vi "Test_IMU_DMP.vi"() -> ()   [LabVIEW 2014]
uses:
  <userlib>/UCSD Robotics Lab/Robotics-Cape/LV/libroboticscape.lvlib
panel:
  out "State":T1(ring)
  out "Timing Block":T2 {"Actual Hz" format="%#_3g"; "Dt" format="%#_4g"; "Average Hz" format="%#_4g"}
  out "Quarternion":T3
  in  "Quarternion On/Off":bool
  in  "Input Prior to Start":T4={"orientation"=112, "IMU_sample_rate "=100, "dmp_interrupt_priority"=98, "Enable Magnetometer"=FALSE} {"dmp_interrupt_priority" min=1 max=99 step=1; "IMU_sample_rate" min=4 max=200; "orientation" items=["ORIENTATION_Z_UP"=136, "ORIENTATION_Z_DOWN"=396, "ORIENTATION_X_UP"=14, "ORIENTATION_X_DOWN"=266, "ORIENTATION_Y_UP"=112, "ORIENTATION_Y_DOWN"=336, "ORIENTATION_X_FORWARD"=133, "ORIENTATION_X_BACK"=161]}
  out "Gryo":T5
  out "Accel":T6
  out "Tait Bryan":T7
  in  "Gyro On/Off":bool
  in  "Accel On/Off":bool
  in  "TaitBryan On/Off":bool
  in  "Compass On/Off":bool
  out "Compass":T8
  in  "stop":bool
  # "Always stop the VI using the rectangular STOP button below, never with the round stopsign (Abort)"
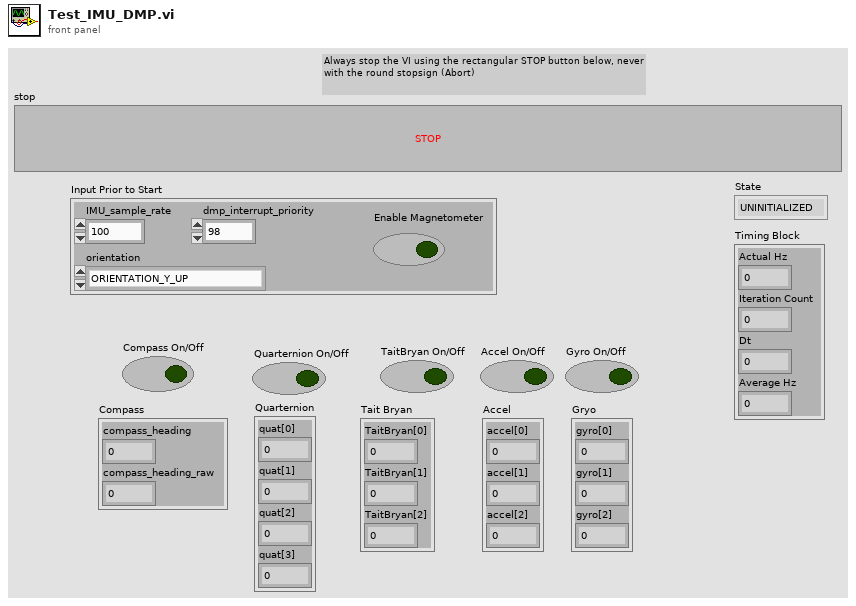
[diagram p1: front panel]
types:
  T1 = enum16{"UNINITIALIZED", "RUNNING", "PAUSED", "EXITING"}
  T2 = cluster{"Actual Hz":dbl, "Iteration Count":dbl, "Dt":dbl, "Average Hz":dbl}
  T3 = cluster{"quat[0]":sgl, "quat[1]":sgl, "quat[2]":sgl, "quat[3]":sgl}
  T4 = cluster{"orientation":u32, "IMU_sample_rate ":i32, "dmp_interrupt_priority":i32, "Enable Magnetometer":bool}
  T5 = cluster{"gyro[0]":sgl, "gyro[1]":sgl, "gyro[2]":sgl}
  T6 = cluster{"accel[0]":sgl, "accel[1]":sgl, "accel[2]":sgl}
  T7 = cluster{"TaitBryan[0]":dbl, "TaitBryan[1]":dbl, "TaitBryan[2]":dbl}
  T8 = cluster{"compass_heading":sgl, "compass_heading_raw":sgl}
  T9 = cluster{"accel[0]":sgl, "accel[1]":sgl, "accel[2]":sgl, "gyro[0]":sgl, "gyro[1]":sgl, "gyro[2]":sgl, "mag[0]":sgl, "mag[1]":sgl, "mag[2]":sgl, "temp":sgl, "raw_gyro[0]":i16, "raw_gyro[1]":i16, "raw_gyro[2]":i16, "raw_accel[0]":i16, "raw_accel[1]":i16, "raw_accel[2]":i16, "accel_to_ms2":sgl, "gyro_to_degs":sgl, "dmp_quat[0]":sgl, "dmp_quat[1]":sgl, "dmp_quat[2]":sgl, "dmp_quat[3]":sgl, "dmp_TaitBryan[0]":sgl, "dmp_TaitBryan[1]":sgl, "dmp_TaitBryan[2]":sgl, "fused_quat[0]":sgl, "fused_quat[1]":sgl, "fused_quat[2]":sgl, "fused_quat[3]":sgl, "fused_TaitBryan[0]":sgl, "fused_TaitBryan[1]":sgl, "fused_TaitBryan[2]":sgl, "compass_heading":sgl, "compass_heading_raw":sgl}
  T10 = enum16{"UNINITIALIZED", "RUNING", "PAUSED", "EXITING"}
  T11 = cluster{"fused_quat[0]":sgl, "fused_quat[1]":sgl, "fused_quat[2]":sgl, "fused_quat[3]":sgl}
  T12 = cluster{"fused_TaitBryan[0]":sgl, "fused_TaitBryan[1]":sgl, "fused_TaitBryan[2]":sgl}
  T13 = cluster{"fused_TaitBryan[0]":dbl, "fused_TaitBryan[1]":dbl, "fused_TaitBryan[2]":dbl}
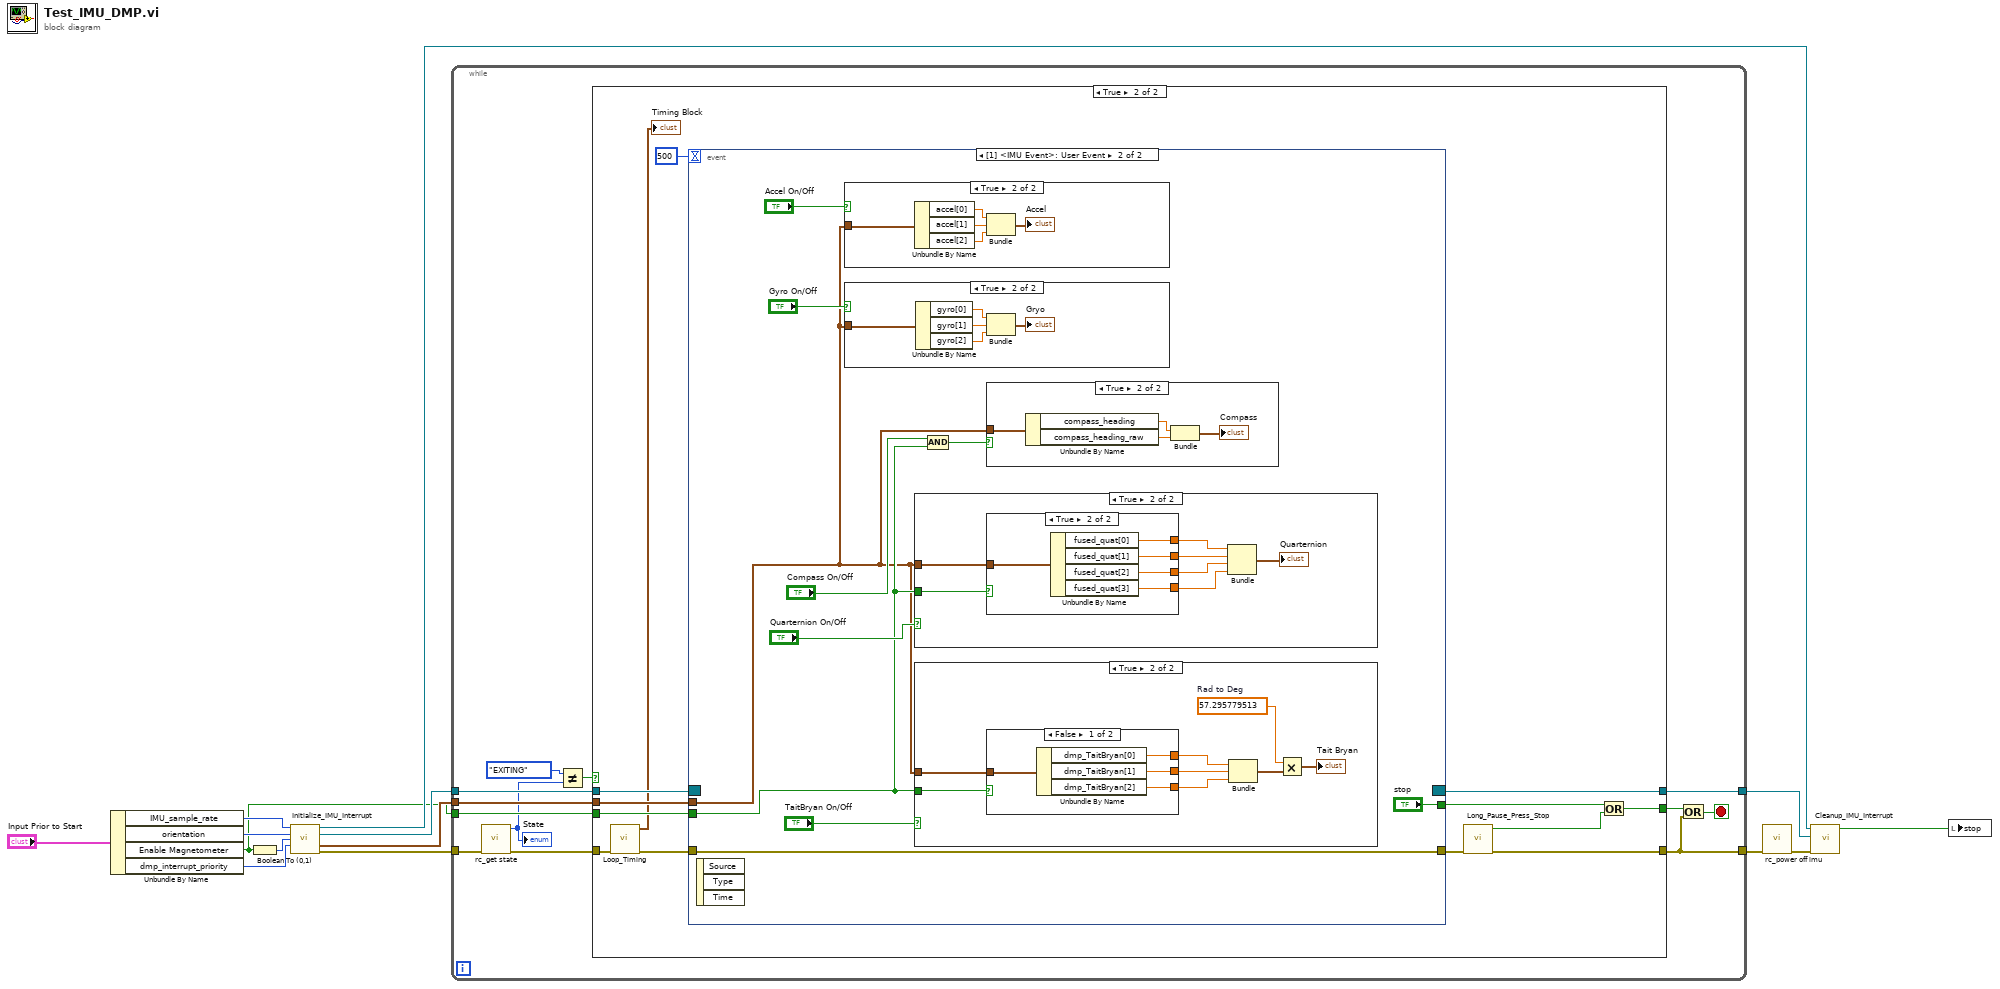
[diagram p0: block diagram]
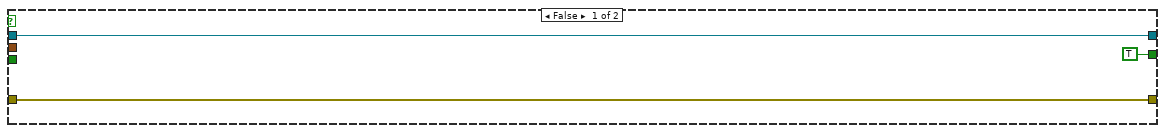
[diagram p2: hidden frame]
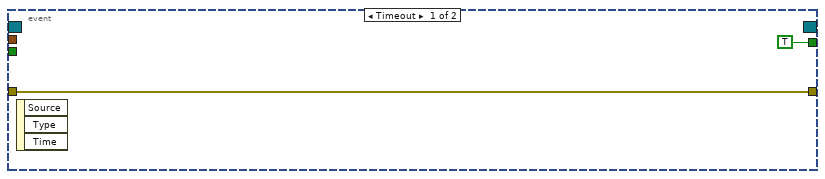
[diagram p3: hidden frame]
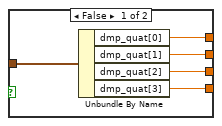
[diagram p5: hidden frame]
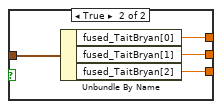
[diagram p9: hidden frame]
diagram:
  n1 = Unbundle By Name("Input Prior to Start") -> ("IMU_sample_rate"=w6:i32, "orientation"=w5:u32, "Enable Magnetometer"=w3:bool, "dmp_interrupt_priority"=w4:i32)
  n2 = Boolean To (0,1)(Boolean=w3) -> (0, 1=w8:i16)
  n3 = call "Initialize_IMU_Interrupt.vi"("dmp_sample_rate"=w6, "orientation"=w5, "enable_magnetometer"=w8, "dmp_interrupt_priority"=w4) -> ("IMU Event"=w12:refnum<user-event>, "Event Registration Refnum"=w14:refnum<event-registration>, "IMU Data"=w10:T9, "error out"=w9:errorcluster)  [unwired: 8 in]
  n4 = while {
    tunnel: w9 -> [w21]
    tunnel: [w26] -> w11
    tunnel: [w24] -> w2
    tunnel: w14 -> [w25]
    tunnel: w10 -> [w22]
    tunnel: w3 -> [w16]
    stop <- w23 stop-if-true
    n5 = call <userlib>:"rc_get state.vi"("error in (no error)"=w21) -> ("error out"=w20:errorcluster, "function return"=w15:u32)  [unwired: 9 in]
    "State" <- w15
    n6 = Not Equal?(x=T10."EXITING" ("State 2"), y=w15) -> (x != y?=w18:bool)
    n7 = case shown="True" w18 {
      tunnel: [w28 w42] -> w26
      tunnel: w25 -> [w28 w40]
      tunnel: [w29 w33] -> w24
      tunnel: w22 -> [_ w39]
      tunnel: w20 -> [w29 w37]
      tunnel: [TRUE ("stop") w30] -> w17
      tunnel: w16 -> [_ w38]
      frame False {
      }
      frame True {
        n8 = call "Loop_Timing.vi"("error in"=w37) -> ("error out"=w36:errorcluster, "Timing Block"=→"Timing Block":T2)  [unwired: 9 in]
        n9 = event shown="[1] <IMU Event>: User Event" {
          selector: w40 -> [_ _]
          dyn-events: [_ _] -> w42
          timeout: 500 -> [_ _]
          tunnel: w36 -> [w44 w54]
          tunnel: [w44 w54] -> w34
          tunnel: w39 -> [_ w46]
          tunnel: w38 -> [_ w47]
          tunnel: [TRUE ("stop") "stop"] -> w32
          event Timeout {
            n10 = event-data() -> ()  [unwired: 1 in, 3 out]
          }
          event User Event {
            n11 = event-data() -> ()  [unwired: 1 in, 3 out]
            n12 = case shown="True" "Accel On/Off" {
              tunnel: w46 -> [_ w81]
              frame False {
              }
              frame True {
                n13 = Unbundle By Name(w81) -> ("accel[0]"=w80:sgl, "accel[1]"=w79:sgl, "accel[2]"=w78:sgl)
                n14 = Bundle("accel[0]"=w80, "accel[1]"=w79, "accel[2]"=w78) -> (→"Accel":T6)  [unwired: 1 in]
              }
            }
            n15 = case shown="True" "Gyro On/Off" {
              tunnel: w46 -> [_ w76]
              frame False {
              }
              frame True {
                n16 = Unbundle By Name(w76) -> ("gyro[0]"=w75:sgl, "gyro[1]"=w74:sgl, "gyro[2]"=w73:sgl)
                n17 = Bundle("gyro[0]"=w75, "gyro[1]"=w74, "gyro[2]"=w73) -> (→"Gryo":T5)  [unwired: 1 in]
              }
            }
            n18 = case shown="True" "Quarternion On/Off" {
              tunnel: w46 -> [_ w61]
              tunnel: w47 -> [_ w55]
              frame False {
              }
              frame True {
                n19 = case shown="True" w55 {
                  tunnel: w61 -> [w66 w71]
                  tunnel: [w65 w70] -> w60
                  tunnel: [w64 w69] -> w59
                  tunnel: [w63 w68] -> w58
                  tunnel: [w62 w67] -> w57
                  frame False {
                    n20 = Unbundle By Name(w66) -> ("dmp_quat[0]"=w65:sgl, "dmp_quat[1]"=w64:sgl, "dmp_quat[2]"=w63:sgl, "dmp_quat[3]"=w62:sgl)
                  }
                  frame True {
                    n21 = Unbundle By Name(w71) -> ("fused_quat[0]"=w70:sgl, "fused_quat[1]"=w69:sgl, "fused_quat[2]"=w68:sgl, "fused_quat[3]"=w67:sgl)
                  }
                }
                n22 = Bundle("fused_quat[0]"=w60, "fused_quat[1]"=w59, "fused_quat[2]"=w58, "fused_quat[3]"=w57) -> (→"Quarternion":T11)  [unwired: 1 in]
              }
            }
            n23 = case shown="True" "TaitBryan On/Off" {
              tunnel: w46 -> [_ w89]
              tunnel: w47 -> [_ w82]
              frame False {
              }
              frame True {
                w84 = 57.295779513  # Rad to Deg
                n24 = case shown="False" w82 {
                  tunnel: w89 -> [w93 w97]
                  tunnel: [w92 w96] -> w88
                  tunnel: [w91 w95] -> w87
                  tunnel: [w90 w94] -> w86
                  frame False {
                    n25 = Unbundle By Name(w93) -> ("dmp_TaitBryan[0]"=w92:sgl, "dmp_TaitBryan[1]"=w91:sgl, "dmp_TaitBryan[2]"=w90:sgl)
                  }
                  frame True {
                    n26 = Unbundle By Name(w97) -> ("fused_TaitBryan[0]"=w96:sgl, "fused_TaitBryan[1]"=w95:sgl, "fused_TaitBryan[2]"=w94:sgl)
                  }
                }
                n27 = Bundle("fused_TaitBryan[0]"=w88, "fused_TaitBryan[1]"=w87, "fused_TaitBryan[2]"=w86) -> (w85:T12)  [unwired: 1 in]
                n28 = Multiply(x=w84, y=w85) -> (x*y=→"Tait Bryan":T13)
              }
            }
            n29 = And(x="Compass On/Off", y=w47) -> (x .and. y?=w50:bool)
            n30 = case shown="True" w50 {
              tunnel: w46 -> [_ w101]
              frame False {
              }
              frame True {
                n31 = Unbundle By Name(w101) -> ("compass_heading"=w100:sgl, "compass_heading_raw"=w99:sgl)
                n32 = Bundle("compass_heading"=w100, "compass_heading_raw"=w99) -> (→"Compass":T8)  [unwired: 1 in]
              }
            }
          }
        }
        n33 = call "Long_Pause_Press_Stop.vi"("error in (no error)"=w34) -> ("error out"=w33:errorcluster, "Stop"=w31:bool)  [unwired: 9 in]
        n34 = Or(x=w32, y=w31) -> (x .or. y?=w30:bool)
      }
    }
    n35 = Or(x=w17, y=w24) -> (x .or. y?=w23:bool)
  }
  n36 = call <userlib>:"rc_power off imu.vi"("error in (no error)"=w2) -> ("error out"=w1:errorcluster)  [unwired: 9 in, 1 out]
  n37 = call "Cleanup_IMU_Interrupt.vi"("error in (no error)"=w1, "Event Registration Refnum 2"=w11, "IMU Event"=w12) -> ("Stop Local Variabl"=w13:bool)  [unwired: 6 in]
  n38 = local write "stop"(w13) -> ()
